vi "OP2_INS1ASSE.vi"(0 "Esito 2 in":cluster{"Si":bool, "No":bool}, 1 "Esito 3 in":cluster{"Si":bool, "No":bool}, 2 "Esito 4 in":cluster{"Si":bool, "No":bool}, 3 "Esito 5 in":cluster{"Si":bool, "No":bool}, 4 "Esito 6 in":cluster{"Si":bool, "No":bool}, 5 "Esito 7 in":cluster{"Si":bool, "No":bool}, 6 "Esito 8 in":cluster{"Si":bool, "No":bool}, 7 "Esito 9 in":cluster{"Si":bool, "No":bool}, 8 "Esito 1 in":cluster{"Si":bool, "No":bool}, 9 "Tasto premuto":T1(array[ring]), 10 "Tipo specifica":string, 12 "Stato in":u16, 14 "Stato out":u16) -> (16 "Dato":string[](array[string]), 17 "ANNULLA PROVA":bool, 18 "Esito 1 out":T2, 19 "i out":i32=1, 20 "Esito 2 out":T2, 21 "Esito 3 out":T2, 22 "Esito 4 out":T2, 23 "Esito 5 out":T2, 24 "Esito 6 out":T2, 25 "Esito 7 out":T2, 26 "Esito 8 out":T2, 27 "Esito 9 out":T2)   [LabVIEW 2022 SP3]
uses:
  Labview/Globali.vi
panel:
  in  "i max":i32
  in  "i":i32=1
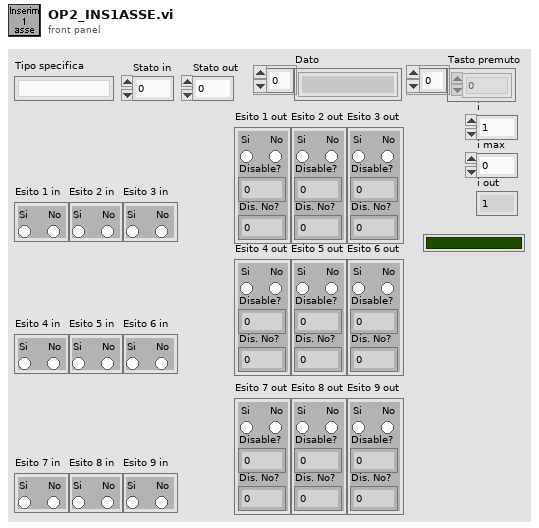
[diagram p1: front panel]
types:
  T1 = enum16{"0", "1", "2", "3", "4", "5", "6", "7", "8", "9", "A", "B", "C", "D", "E", "F", "G", "H", "I", "J", "K", "L", "M", "N", "O", "P", "Q", "R", "S", "T", "U", "V", "W", "X", "Y", "Z", "F1", "F2", "F3", "F4", "F5", "F6", "F7", "F8", "F9", "F10", "F11", "F12", "F13", "F14", "F15", "ADD", "BACK", "BACKSLASH", "CAPITAL", "COMMA", "DECIMAL", "DELETE", "DIVIDE", "DOWN", "END", "EQUALS", "ESCAPE", "GRAVE (`)", "HOME", "INSERT", "LBRACKET", "LCONTROL", "LEFT", "L ALT", "LSHIFT", "LWIN", "MINUS", "MULTIPLY", "NEXT", "NUMLOCK", "NUMPAD_0", "NUMPAD_1", "NUMPAD_2", "NUMPAD_3", "NUMPAD_4", "NUMPAD_5", "NUMPAD_6", "NUMPAD_7", "NUMPAD_8", "NUMPAD_9", "PAUSE", "PERIOD", "PRIOR (PG UP)", "RBRACKET", "RCONTROL", "RETURN", "RIGHT", "R ALT", "RSHIFT", "RWIN", "SCROLL", "SEMICOLON", "SLASH", "SPACE", "SUBTRACT", "TAB", "UP", "ENTER (num pad)", "' (quote)"}[]
  T2 = cluster{"Disable?":i16, "Si":bool, "No":bool, "Dis. No?":i16}
  T3 = cluster{"Esito 1 out":cluster{"Disable?":i16, "Si":bool, "No":bool, "Dis. No?":i16}, "Esito 2 out":cluster{"Disable?":i16, "Si":bool, "No":bool, "Dis. No?":i16}, "Esito 3 out":cluster{"Disable?":i16, "Si":bool, "No":bool, "Dis. No?":i16}, "Esito 4 out":cluster{"Disable?":i16, "Si":bool, "No":bool, "Dis. No?":i16}, "Esito 5 out":cluster{"Disable?":i16, "Si":bool, "No":bool, "Dis. No?":i16}, "Esito 6 out":cluster{"Disable?":i16, "Si":bool, "No":bool, "Dis. No?":i16}, "Esito 7 out":cluster{"Disable?":i16, "Si":bool, "No":bool, "Dis. No?":i16}, "Esito 8 out":cluster{"Disable?":i16, "Si":bool, "No":bool, "Dis. No?":i16}, "Esito 9 out":cluster{"Disable?":i16, "Si":bool, "No":bool, "Dis. No?":i16}}
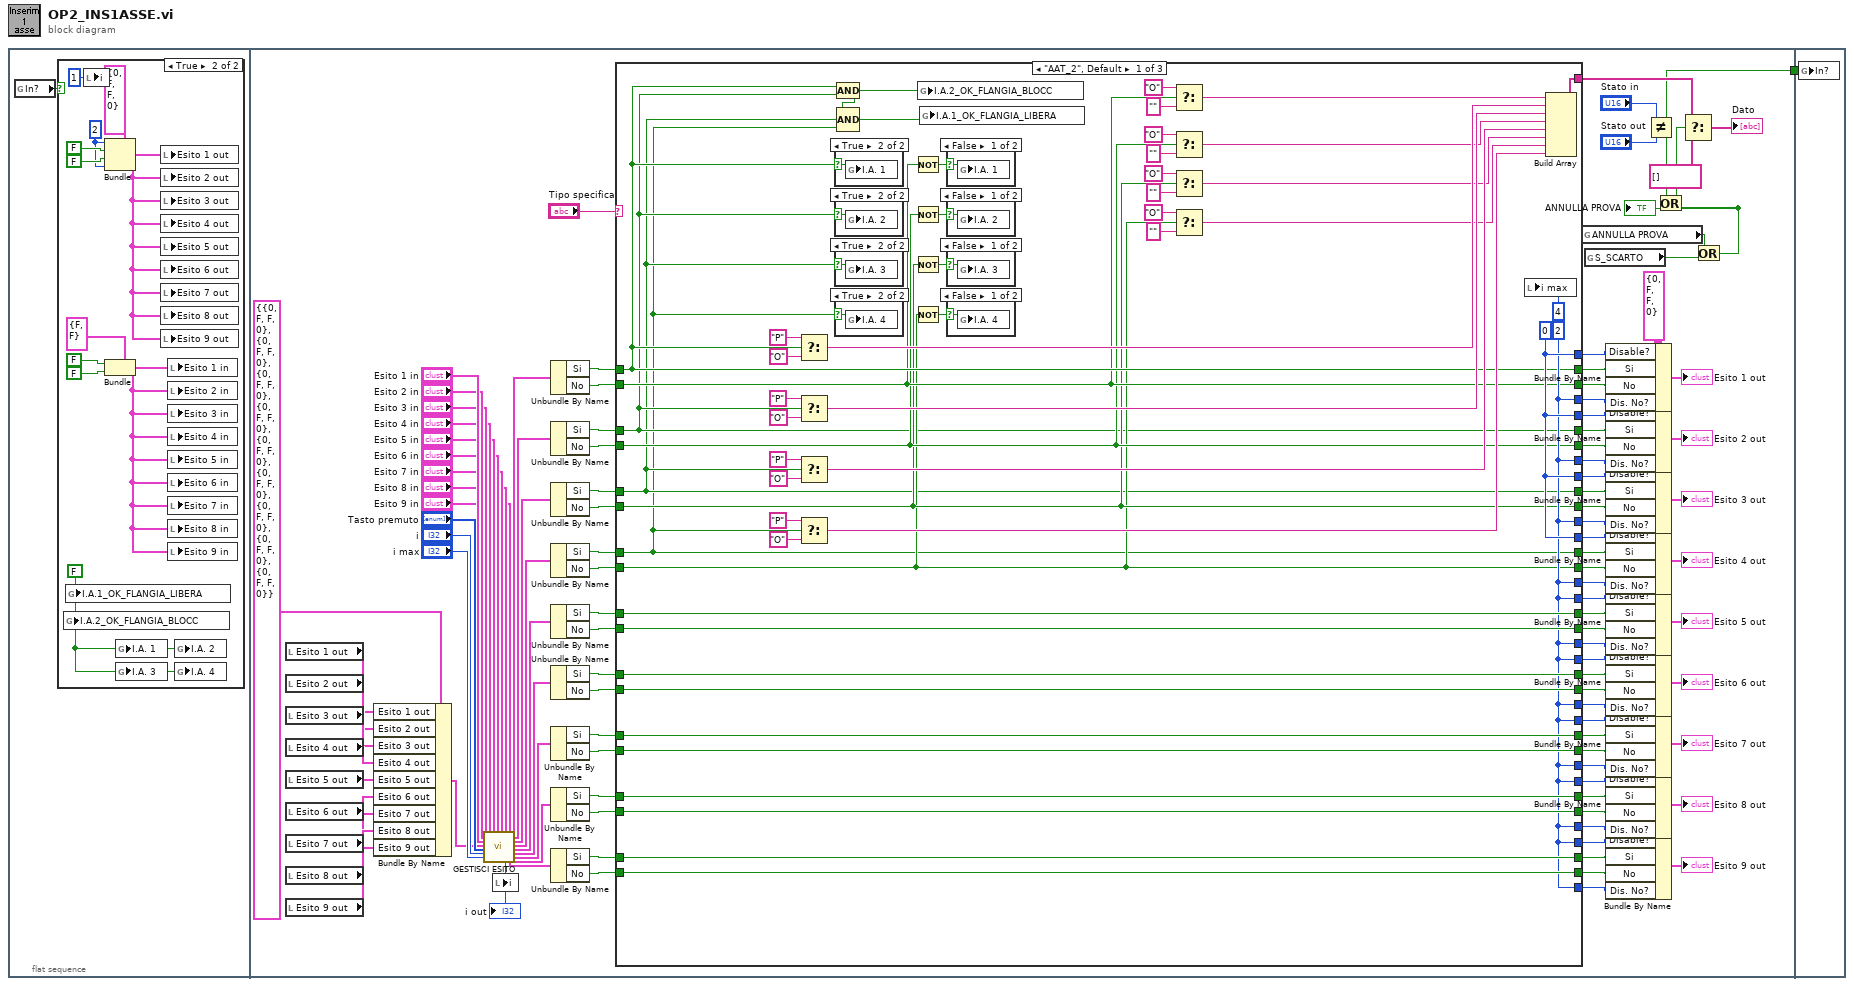
[diagram p0: block diagram]
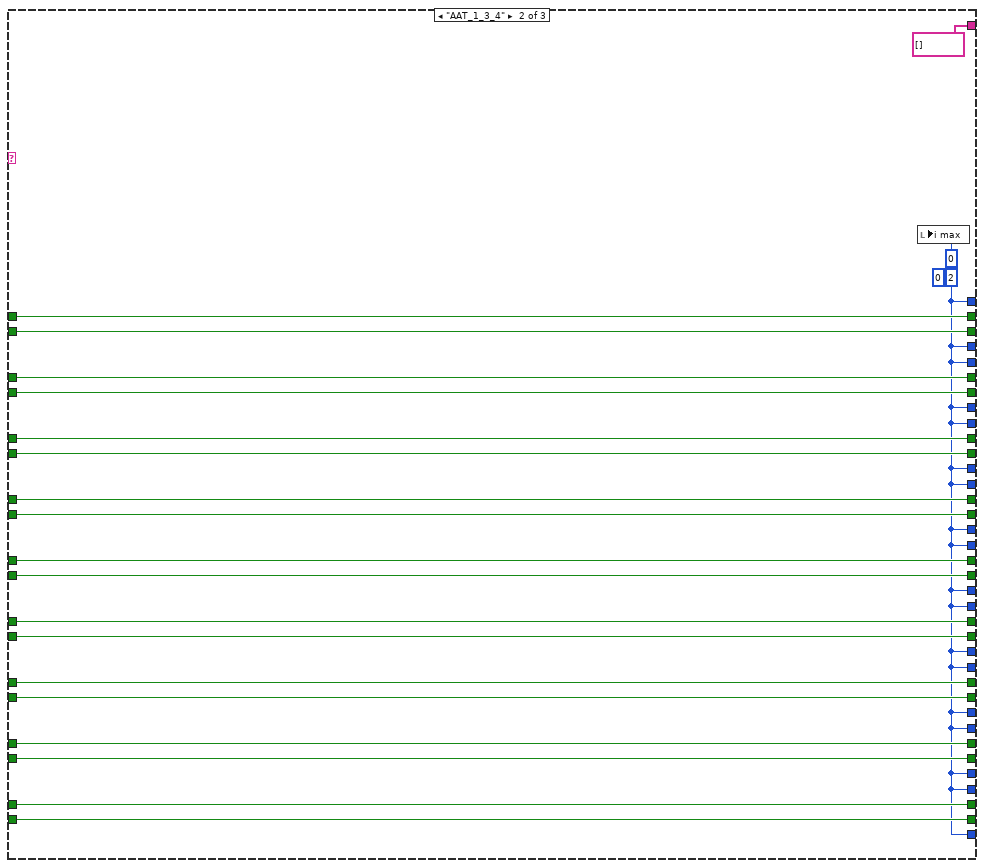
[diagram p11: hidden frame]
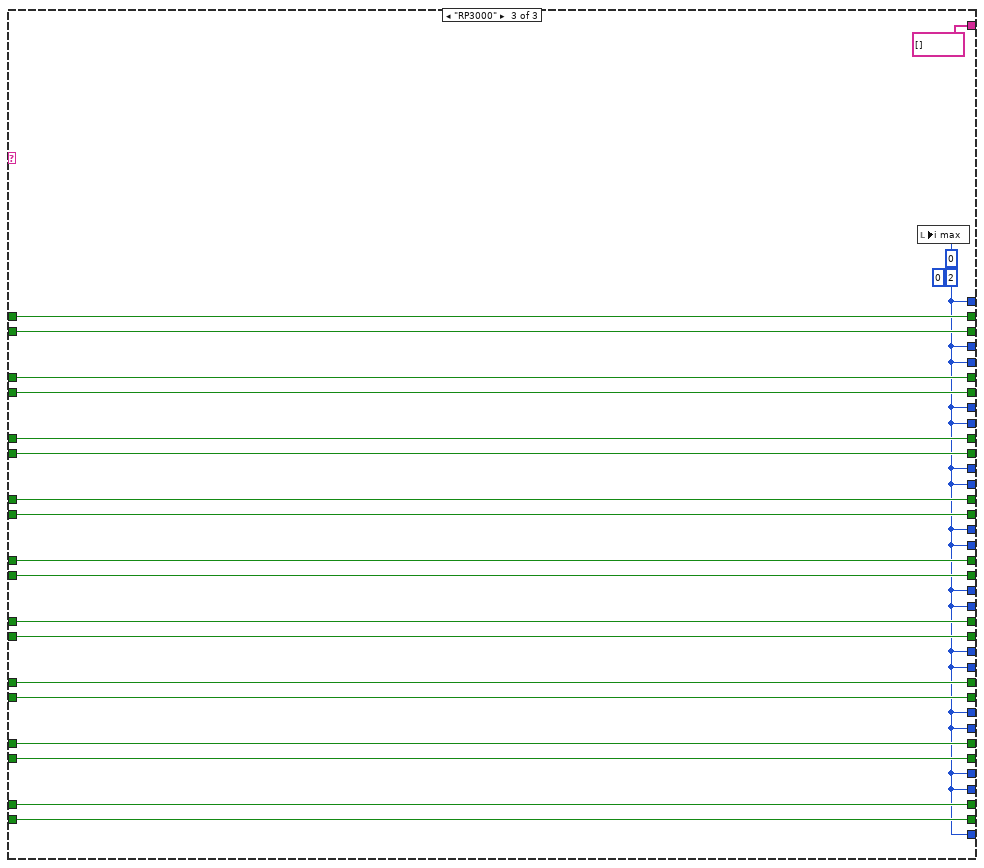
[diagram p12: hidden frame]
diagram:
  n1 = flat-sequence {
    tunnel: [w18] -> w1
    tunnel: w1 -> [w224]
    frame #0 {
      n2 = global read "Globali.vi" "In?"() -> (w2:bool)
      n3 = case shown="True" w2 {
        frame False {
        }
        frame True {
          w3 = FALSE
          w10 = i16 2 ("Disable?")
          n4 = global write "Globali.vi" "I.A.2_OK_FLANGIA_BLOCC"(w3) -> ()
          n5 = global write "Globali.vi" "I.A.1_OK_FLANGIA_LIBERA"(w3) -> ()
          n6 = local write "i"(1 ("i")) -> ()
          n7 = Bundle(cluster=T2 {"Disable?"=0, "Si"=FALSE, "No"=FALSE, "Dis. No?"=0} ("Esito 1 out"), "Disable?"=w10, "Si"=FALSE, "No"=FALSE, "Dis. No?"=w10) -> (w9:T2)
          n8 = Bundle(cluster=cluster{"Si":bool, "No":bool} {"Si"=FALSE, "No"=FALSE} ("Esito 1 in"), "Si"=FALSE, "No"=FALSE) -> (w7:cluster{"Si":bool, "No":bool})
          n9 = global write "Globali.vi" "I.A. 1"(w3) -> ()
          n10 = global write "Globali.vi" "I.A. 3"(w3) -> ()
          n11 = local write "Esito 1 out"(w9) -> ()
          n12 = local write "Esito 2 out"(w9) -> ()
          n13 = local write "Esito 3 out"(w9) -> ()
          n14 = local write "Esito 4 out"(w9) -> ()
          n15 = local write "Esito 5 out"(w9) -> ()
          n16 = local write "Esito 6 out"(w9) -> ()
          n17 = local write "Esito 7 out"(w9) -> ()
          n18 = local write "Esito 8 out"(w9) -> ()
          n19 = local write "Esito 9 out"(w9) -> ()
          n20 = local write "Esito 1 in"(w7) -> ()
          n21 = local write "Esito 2 in"(w7) -> ()
          n22 = local write "Esito 3 in"(w7) -> ()
          n23 = local write "Esito 4 in"(w7) -> ()
          n24 = local write "Esito 5 in"(w7) -> ()
          n25 = local write "Esito 6 in"(w7) -> ()
          n26 = local write "Esito 7 in"(w7) -> ()
          n27 = local write "Esito 8 in"(w7) -> ()
          n28 = local write "Esito 9 in"(w7) -> ()
          n29 = global write "Globali.vi" "I.A. 2"(w3) -> ()
          n30 = global write "Globali.vi" "I.A. 4"(w3) -> ()
        }
      }
    }
    frame #1 {
      w61 = T2 {"Disable?"=0, "Si"=FALSE, "No"=FALSE, "Dis. No?"=0} ("Esito 1 out")
      n31 = local read "Esito 1 out"() -> (w39:T2)
      n32 = local read "Esito 2 out"() -> (w40:T2)
      n33 = local read "Esito 3 out"() -> (w41:T2)
      n34 = local read "Esito 4 out"() -> (w42:T2)
      n35 = local read "Esito 5 out"() -> (w43:T2)
      n36 = local read "Esito 6 out"() -> (w44:T2)
      n37 = local read "Esito 7 out"() -> (w45:T2)
      n38 = local read "Esito 8 out"() -> (w46:T2)
      n39 = local read "Esito 9 out"() -> (w47:T2)
      n40 = Bundle By Name(cluster=T3 {"Esito 1 out"={"Disable?"=0, "Si"=FALSE, "No"=FALSE, "Dis. No?"=0}, "Esito 2 out"={"Disable?"=0, "Si"=FALSE, "No"=FALSE, "Dis. No?"=0}, "Esito 3 out"={"Disable?"=0, "Si"=FALSE, "No"=FALSE, "Dis. No?"=0}, "Esito 4 out"={"Disable?"=0, "Si"=FALSE, "No"=FALSE, "Dis. No?"=0}, "Esito 5 out"={"Disable?"=0, "Si"=FALSE, "No"=FALSE, "Dis. No?"=0}, "Esito 6 out"={"Disable?"=0, "Si"=FALSE, "No"=FALSE, "Dis. No?"=0}, "Esito 7 out"={"Disable?"=0, "Si"=FALSE, "No"=FALSE, "Dis. No?"=0}, "Esito 8 out"={"Disable?"=0, "Si"=FALSE, "No"=FALSE, "Dis. No?"=0}, "Esito 9 out"={"Disable?"=0, "Si"=FALSE, "No"=FALSE, "Dis. No?"=0}} ("Cluster"), "Esito 1 out"=w39, "Esito 2 out"=w40, "Esito 3 out"=w41, "Esito 4 out"=w42, "Esito 5 out"=w43, "Esito 6 out"=w44, "Esito 7 out"=w45, "Esito 8 out"=w46, "Esito 9 out"=w47) -> (w48:T3)
      n41 = call "GESTISCI ESITO.vi"("Esito 3 in"="Esito 3 in", "Esito 2 in"="Esito 2 in", "Esito 1 in"="Esito 1 in", "Cluster"=w48, "Tasto premuto"="Tasto premuto", "i in"="i", "i max"="i max", "Esito 4 in"="Esito 4 in", "Esito 5 in"="Esito 5 in", "Esito 6 in"="Esito 6 in", "Esito 7 in"="Esito 7 in", "Esito 8 in"="Esito 8 in", "Esito 9 in"="Esito 9 in") -> ("i out"=w19:i32, "Esito 9 in 2"=w37:cluster{"Si":bool, "No":bool}, "Esito 1 in 2"=w36:cluster{"Si":bool, "No":bool}, "Esito 2 in 2"=w35:cluster{"Si":bool, "No":bool}, "Esito 3 in 2"=w34:cluster{"Si":bool, "No":bool}, "Esito 4 in 2"=w33:cluster{"Si":bool, "No":bool}, "Esito 5 in 2"=w32:cluster{"Si":bool, "No":bool}, "Esito 6 in 2"=w31:cluster{"Si":bool, "No":bool}, "Esito 7 in 2"=w30:cluster{"Si":bool, "No":bool}, "Esito 8 in 2"=w29:cluster{"Si":bool, "No":bool})  [unwired: 5 in]
      "i out" <- w19
      n42 = local write "i"(w19) -> ()
      n43 = Unbundle By Name(w36) -> ("Si"=w85:bool, "No"=w84:bool)
      n44 = Unbundle By Name(w35) -> ("Si"=w68:bool, "No"=w69:bool)
      n45 = Unbundle By Name(w34) -> ("Si"=w70:bool, "No"=w71:bool)
      n46 = Unbundle By Name(w33) -> ("Si"=w72:bool, "No"=w73:bool)
      n47 = Unbundle By Name(w32) -> ("Si"=w74:bool, "No"=w75:bool)
      n48 = Unbundle By Name(w31) -> ("Si"=w76:bool, "No"=w77:bool)
      n49 = Unbundle By Name(w30) -> ("Si"=w78:bool, "No"=w79:bool)
      n50 = Unbundle By Name(w29) -> ("Si"=w80:bool, "No"=w81:bool)
      n51 = Unbundle By Name(w37) -> ("Si"=w82:bool, "No"=w83:bool)
      n52 = case shown="\"AAT_2\", Default" "Tipo specifica" {
        tunnel: [w158 string[] [] ("Dato") string[] [] ("Dato")] -> w65
        tunnel: [w135 w184 w205] -> w112
        tunnel: [w135 w184 w205] -> w111
        tunnel: [w135 w184 w205] -> w110
        tunnel: [w135 w184 w205] -> w109
        tunnel: [w134 w184 w205] -> w108
        tunnel: [w134 w184 w205] -> w107
        tunnel: [w134 w184 w205] -> w106
        tunnel: [w134 w184 w205] -> w105
        tunnel: [w134 w184 w205] -> w104
        tunnel: [w133 w185 w206] -> w103
        tunnel: [w131 w192 w213] -> w102
        tunnel: [w124 w191 w212] -> w101
        tunnel: [w127 w193 w214] -> w100
        tunnel: [w123 w186 w207] -> w99
        tunnel: [w126 w202 w223] -> w98
        tunnel: [w122 w187 w208] -> w97
        tunnel: [w125 w201 w222] -> w96
        tunnel: [w154 w190 w211] -> w95
        tunnel: [w173 w200 w221] -> w94
        tunnel: [w153 w189 w210] -> w93
        tunnel: [w172 w199 w220] -> w92
        tunnel: [w152 w188 w209] -> w91
        tunnel: [w171 w198 w219] -> w90
        tunnel: [w170 w197 w218] -> w89
        tunnel: [w169 w196 w217] -> w88
        tunnel: [w168 w195 w216] -> w87
        tunnel: [w167 w194 w215] -> w86
        tunnel: w85 -> [w133 w185 w206]
        tunnel: w84 -> [w131 w192 w213]
        tunnel: w83 -> [w167 w194 w215]
        tunnel: w82 -> [w168 w195 w216]
        tunnel: w81 -> [w169 w196 w217]
        tunnel: w80 -> [w170 w197 w218]
        tunnel: w79 -> [w171 w198 w219]
        tunnel: w78 -> [w152 w188 w209]
        tunnel: w77 -> [w172 w199 w220]
        tunnel: w76 -> [w153 w189 w210]
        tunnel: w75 -> [w173 w200 w221]
        tunnel: w74 -> [w154 w190 w211]
        tunnel: w73 -> [w125 w201 w222]
        tunnel: w72 -> [w122 w187 w208]
        tunnel: w71 -> [w126 w202 w223]
        tunnel: w70 -> [w123 w186 w207]
        tunnel: w69 -> [w127 w193 w214]
        tunnel: w68 -> [w124 w191 w212]
        tunnel: [w134 w184 w205] -> w60
        tunnel: [w134 w184 w205] -> w59
        tunnel: [w134 w184 w205] -> w58
        tunnel: [w134 w184 w205] -> w57
        tunnel: [w134 w184 w205] -> w56
        tunnel: [w134 w184 w205] -> w55
        tunnel: [w134 w184 w205] -> w54
        tunnel: [w134 w184 w205] -> w53
        tunnel: [w134 w184 w205] -> w52
        frame "AAT_2", Default {
          w134 = 2
          w135 = 0
          n53 = Select(t="P", s=w133, f="O") -> (s? t:f=w148:string)
          n54 = Select(t="P", s=w124, f="O") -> (s? t:f=w155:string)
          n55 = Select(t="P", s=w123, f="O") -> (s? t:f=w156:string)
          n56 = Select(t="P", s=w122, f="O") -> (s? t:f=w157:string)
          n57 = case shown="True" w133 {
            selector: w133 -> [_ w181]
            frame False {
            }
            frame True {
              n58 = global write "Globali.vi" "I.A. 1"(w181) -> ()
            }
          }
          n59 = case shown="True" w124 {
            selector: w124 -> [_ w179]
            frame False {
            }
            frame True {
              n60 = global write "Globali.vi" "I.A. 2"(w179) -> ()
            }
          }
          n61 = case shown="True" w123 {
            selector: w123 -> [_ w177]
            frame False {
            }
            frame True {
              n62 = global write "Globali.vi" "I.A. 3"(w177) -> ()
            }
          }
          n63 = case shown="True" w122 {
            selector: w122 -> [_ w175]
            frame False {
            }
            frame True {
              n64 = global write "Globali.vi" "I.A. 4"(w175) -> ()
            }
          }
          n65 = Compound Arithmetic op=AND(w133, w124) -> (w136:bool)
          n66 = Compound Arithmetic op=AND(w136, w123, w122) -> (w151:bool)
          n67 = Not(x=w131) -> (.not. x?=w132:bool)
          n68 = Not(x=w127) -> (.not. x?=w130:bool)
          n69 = Not(x=w126) -> (.not. x?=w129:bool)
          n70 = Not(x=w125) -> (.not. x?=w128:bool)
          n71 = global write "Globali.vi" "I.A.2_OK_FLANGIA_BLOCC"(w136) -> ()
          n72 = global write "Globali.vi" "I.A.1_OK_FLANGIA_LIBERA"(w151) -> ()
          n73 = case shown="False" w132 {
            selector: w132 -> [w180 _]
            frame False {
              n74 = global write "Globali.vi" "I.A. 1"(w180) -> ()
            }
            frame True {
            }
          }
          n75 = case shown="False" w130 {
            selector: w130 -> [w178 _]
            frame False {
              n76 = global write "Globali.vi" "I.A. 2"(w178) -> ()
            }
            frame True {
            }
          }
          n77 = case shown="False" w129 {
            selector: w129 -> [w176 _]
            frame False {
              n78 = global write "Globali.vi" "I.A. 3"(w176) -> ()
            }
            frame True {
            }
          }
          n79 = case shown="False" w128 {
            selector: w128 -> [w174 _]
            frame False {
              n80 = global write "Globali.vi" "I.A. 4"(w174) -> ()
            }
            frame True {
            }
          }
          n81 = Select(t="O", s=w131, f="") -> (s? t:f=w147:string)
          n82 = Select(t="O", s=w127, f="") -> (s? t:f=w144:string)
          n83 = Select(t="O", s=w126, f="") -> (s? t:f=w139:string)
          n84 = Select(t="O", s=w125, f="") -> (s? t:f=w138:string)
          n85 = local write "i max"(4) -> ()
          n86 = Build Array(w147, w148, w155, w144, w156, w139, w138, w157) -> (w158:string[])
        }
        frame "AAT_1_3_4" {
          w184 = 2
          (unwired) 0
          n87 = local write "i max"(0) -> ()
        }
        frame "RP3000" {
          w205 = 2
          (unwired) 0
          n88 = local write "i max"(0) -> ()
        }
      }
      n89 = global read "Globali.vi" "ANNULLA PROVA"() -> (w16:bool)
      n90 = global read "Globali.vi" "S_SCARTO"() -> (w15:bool)
      n91 = Bundle By Name(cluster=w61, "Disable?"=w112, "Si"=w103, "No"=w102, "Dis. No?"=w60) -> (→"Esito 1 out":T2)
      n92 = Bundle By Name(cluster=w61, "Disable?"=w111, "Si"=w101, "No"=w100, "Dis. No?"=w59) -> (→"Esito 2 out":T2)
      n93 = Bundle By Name(cluster=w61, "Disable?"=w110, "Si"=w99, "No"=w98, "Dis. No?"=w58) -> (→"Esito 3 out":T2)
      n94 = Bundle By Name(cluster=w61, "Disable?"=w109, "Si"=w97, "No"=w96, "Dis. No?"=w57) -> (→"Esito 4 out":T2)
      n95 = Bundle By Name(cluster=w61, "Disable?"=w108, "Si"=w95, "No"=w94, "Dis. No?"=w56) -> (→"Esito 5 out":T2)
      n96 = Bundle By Name(cluster=w61, "Disable?"=w107, "Si"=w93, "No"=w92, "Dis. No?"=w55) -> (→"Esito 6 out":T2)
      n97 = Bundle By Name(cluster=w61, "Disable?"=w106, "Si"=w91, "No"=w90, "Dis. No?"=w54) -> (→"Esito 7 out":T2)
      n98 = Bundle By Name(cluster=w61, "Disable?"=w105, "Si"=w89, "No"=w88, "Dis. No?"=w53) -> (→"Esito 8 out":T2)
      n99 = Bundle By Name(cluster=w61, "Disable?"=w104, "Si"=w87, "No"=w86, "Dis. No?"=w52) -> (→"Esito 9 out":T2)
      n100 = Not Equal?(x="Stato in", y="Stato out") -> (x != y?=w18:bool)
      n101 = Or(x=w16, y=w15) -> (x .or. y?=w14:bool)
      "ANNULLA PROVA" <- w14
      n102 = Or(x=w18, y=w14) -> (x .or. y?=w17:bool)
      n103 = Select(t=w65, s=w17, f=string[] [] ("Dato")) -> (s? t:f=→"Dato":string[])
    }
    frame #2 {
      n104 = global write "Globali.vi" "In?"(w224) -> ()
    }
  }
